vi "Get Minimum LabVIEW Version.vi"(8 "error in":errorcluster, 11 "9210 in":refnum<class "9210.lvclass">) -> (0 "error out":errorcluster, 2 "Minimum LabVIEW Version":i32, 3 "9210 out":refnum<class "9210.lvclass">)   [LabVIEW 2017, in "Modules.lvlib" / "9210.lvclass"]
uses:
  9210.lvclass
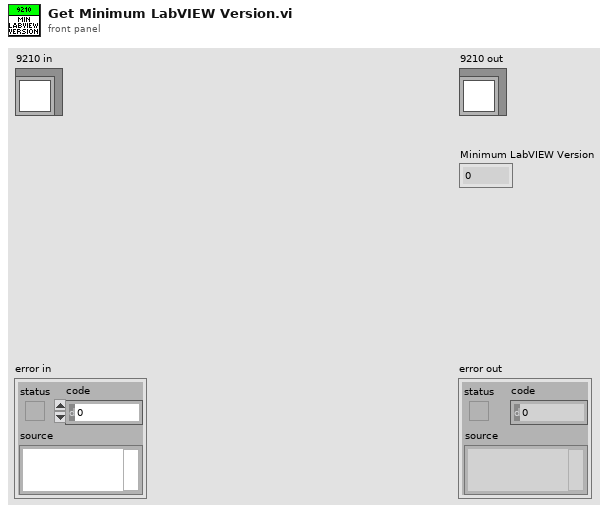
[diagram p1: front panel]
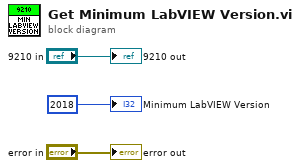
[diagram p0: block diagram]
diagram:
  "error out" <- "error in"
  "9210 out" <- "9210 in"
  "Minimum LabVIEW Version" <- 2018 ("Minimum LabVIEW Version")
